vi "GetSponsorMid.vi"(7 "LabVIEW Web Service Request":refnum<class "Web Request.lvclass">) -> ()   [LabVIEW 2013]
uses:
  <vilib>/wsapi/Web Request.lvclass
panel:
  # "Use the Web Service Request input terminal to call the VIs on the Web Services palette. Do not remove it from the connector pane unless you don't need access to the palette."
  # "Each additional control wired to the connector pane will be available as an input in the URL. To include an indicator in terminal-mode output (the default setting), it must also be wired to the connector pane."
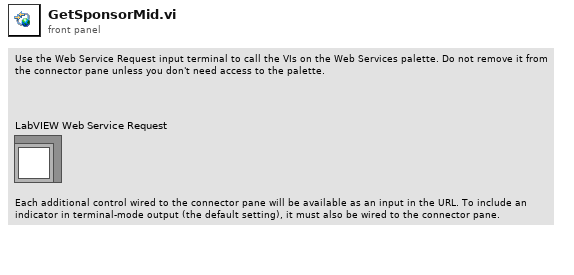
[diagram p1: front panel]
types:
  T1 = typedef "imagedata.ctl" = cluster{"image type":i32, "image depth":i32, "image":u8[], "mask":u8[], "colors":u32[], "Rectangle":cluster{"left":i16, "top":i16, "right":i16, "bottom":i16}}
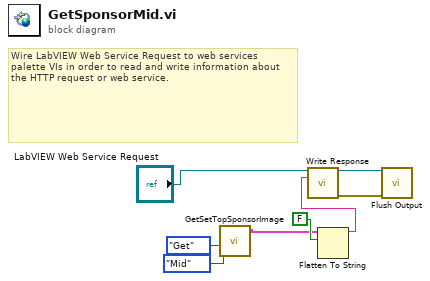
[diagram p0: block diagram]
diagram:
  # "Wire LabVIEW Web Service Request to web services palette VIs in order to read and write information about the HTTP request or web service."
  n1 = call "GetSetTopSponsorImage.vi"("Which"=enum16{"Low", "Mid", "Top"}."Mid", "Get/Set"=enum16{"Get", "Set"}."Get") -> ("image data out"=w1:T1)  [unwired: 9 in]
  n2 = Flatten To String(anything=w1, prepend array or string size? (T)=FALSE) -> (data string=w4:string)  [unwired: 2 in, 2 out]
  n3 = call <vilib>:"Write Response.vi"("LabVIEW Web Service Request"="LabVIEW Web Service Request", "response string"=w4) -> ("LabVIEW Web Service Request out"=w8:refnum<class "Web Request.lvclass">, "error out"=w7:errorcluster)  [unwired: 12 in]
  n4 = call <vilib>:"Flush Output.vi"("LabVIEW Web Service Request"=w8, "error in (no error)"=w7) -> ()  [unwired: 12 in, 2 out]
